vi "barcode.vi"(10 "stop":bool, 11 "Session In":T2) -> (1 "Image":T1(plugin-control), 2 "Boolean":bool, 3 "Data":string)   [LabVIEW 2019]
uses:
  <vilib>/userdefined/High Color/IMAQdx.ctl
  <vilib>/vision/driver/NI_Vision_Acquisition_Software.lvlib
  <vilib>/vision/NI_Vision_Development_Module.lvlib
panel:
  out "error out 5":errorcluster
  out "error out 4":errorcluster
  out "error out 3":errorcluster
  out "error out 2":errorcluster
  out "error out":errorcluster
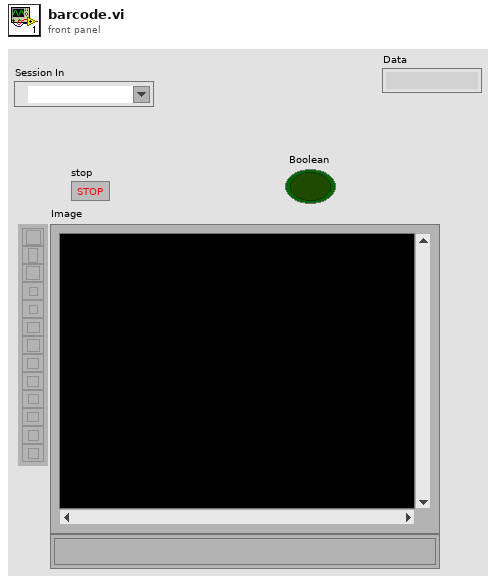
[diagram p1: front panel]
types:
  T1 = typedef "IMAQ Image.ctl" = refnum<image>
  T2 = typedef "IMAQdx.ctl" = refnum<k21>
  T3 = typedef "Image Type" = u32
  T4 = cluster{"Data":string, "Special Char 1":string, "Special Char 2":string, "Checksum(s)":string, "Barcode Type":u32, "Confidence Level":sgl, "Bounding Box":cluster{"x":sgl, "y":sgl}[]}[]
  T5 = cluster{"Data":string, "Special Char 1":string, "Special Char 2":string, "Checksum(s)":string, "Barcode Type":u32, "Confidence Level":sgl, "Bounding Box":cluster{"x":sgl, "y":sgl}[]}
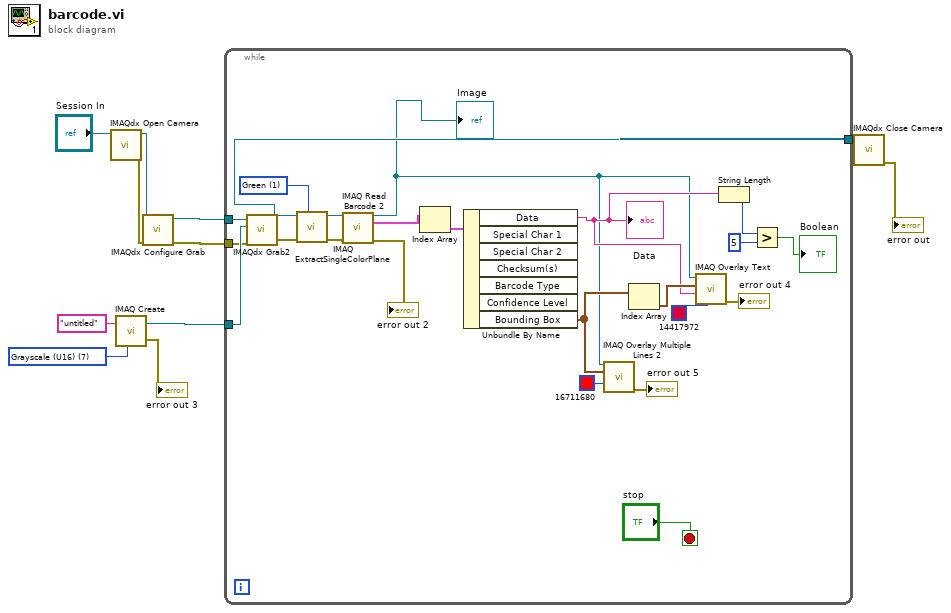
[diagram p0: block diagram]
diagram:
  w1 = T3 7 items=["Grayscale (U8)", "Grayscale (I16)", "Grayscale (SGL)", "Complex (CSG)", "RGB (U32)", "HSL (U32)", "RGB (U64)", "Grayscale (U16)"] ("Image Type")
  n1 = call <vilib>:"IMAQdx Open Camera.vi"("Session In"="Session In") -> ("error out"=w9:errorcluster, "Session Out"=w10:T2)  [unwired: 9 in]
  n2 = call "IMAQ Create"("Image Name"="untitled", "Image Type"=w1) -> ("New Image"=w6:T1, "error out"=→"error out 3":errorcluster)  [unwired: 3 in]
  n3 = call <vilib>:"IMAQdx Configure Grab.vi"("error in"=w9, "Session In"=w10) -> ("error out"=w3:errorcluster, "Session Out"=w7:T2)  [unwired: 8 in]
  n4 = while {
    tunnel: w7 -> [w34]
    tunnel: w6 -> [w35]
    tunnel: [w13] -> w4
    tunnel: w3 -> [w32]
    stop <- "stop" stop-if-true
    w14 = 1 items=["Red", "Green", "Blue", "Hue", "Saturation", "Luminance", "Value", "Intensity"] ("Color Plane")
    n5 = call <vilib>:"IMAQdx Grab2.vi"("error in"=w32, "Image In"=w35, "Session In"=w34) -> ("error out"=w15:errorcluster, "Image Out"=w18:T1, "Session Out"=w13:T2)  [unwired: 5 in, 1 out]
    n6 = call "IMAQ ExtractSingleColorPlane"("Color Plane"=w14, "error in (no error)"=w15, "Image Src"=w18) -> ("error out"=w16:errorcluster, "Image Dst Out"=w17:T1)  [unwired: 7 in]
    n7 = call "IMAQ Read Barcode 2"("Image"=w17, "error in (no error)"=w16) -> ("Image (duplicate)"=w12:T1, "Barcodes"=w30:T4, "error out"=→"error out 2":errorcluster)  [unwired: 9 in, 2 out]
    "Image" <- w12
    n8 = Index Array(array=w30) -> (element=w29:T5)  [unwired: 1 in]
    n9 = Unbundle By Name(w29) -> ("Data"=w22:string, "Bounding Box"=w25:cluster{"x":sgl, "y":sgl}[])  [unwired: 5 out]
    "Data" <- w22
    n10 = call "IMAQ Overlay Multiple Lines 2"("Image"=w12, "Line End Points"=w25, "Color"=u32 16711680) -> ("error out"=→"error out 5":errorcluster)  [unwired: 11 in, 1 out]
    n11 = Index Array(array=w25) -> (element=w28:cluster{"x":sgl, "y":sgl})  [unwired: 1 in]
    n12 = call "IMAQ Overlay Text"("Text Color (black)"=u32 14417972, "String"=w22, "Origin"=w28, "Image"=w12) -> ("error out"=→"error out 4":errorcluster)  [unwired: 6 in, 1 out]
    n13 = String Length(string=w22) -> (length=w21:i32)
    n14 = Greater?(x=w21, y=5) -> (0:→"Boolean":bool)
  }
  n15 = call <vilib>:"IMAQdx Close Camera.vi"("Session In"=w4) -> ("error out"=→"error out":errorcluster)  [unwired: 10 in]
